vi "Teleop.vi"(10 "Match Info":T1={"Autonomous Elapsed Seconds"=0.0, "TeleOp Elapsed Seconds"=0.0, "Disabled Elapsed Seconds"=0.0, "Visited Autonomous"=FALSE, "Visited TeleOp"=FALSE, "Visited Disabled"=FALSE, "Autonomous Settings"={"Autonomous Style"=enum."Independent", "VI Refnum"=refnum}}, 11 "Call Context":T2) -> ()   [LabVIEW 2013]
doc: "This VI is called for each TeleOp packet received from the DS where the robot is not disabled. It is often used to read from the joysticks and update I/O or to update setpoints for timed control loops. It should complete and return within 20 milliseconds or it may miss DS packets."
uses:
  <vilib>/Rock Robotics/WPI/DriverStation/WPI_DriverStationDerivedRobotMode.ctl
  <vilib>/Rock Robotics/WPI/DriverStation/WPI_DriverStationMatch Info.ctl
  <vilib>/Rock Robotics/WPI/Relay/WPI_RelayValue.ctl
  <vilib>/Rock Robotics/WPI/Solenoid/WPI_SolenoidValue.ctl
  Robot Global Data.vi
  <vilib>/Rock Robotics/WPI/Solenoid/WPI_SolenoidSetEnum.vi
  <vilib>/Rock Robotics/WPI/Joystick/WPI_JoystickGetSetRefNum.vi
  <vilib>/Rock Robotics/WPI/RobotDrive/WPI_RobotDriveGetSetRefNum.vi
panel:
  out "Numeric 1":dbl(slide) scale=0.0..100.0
  out "Boolean 2":bool
  out "Boolean 1":bool
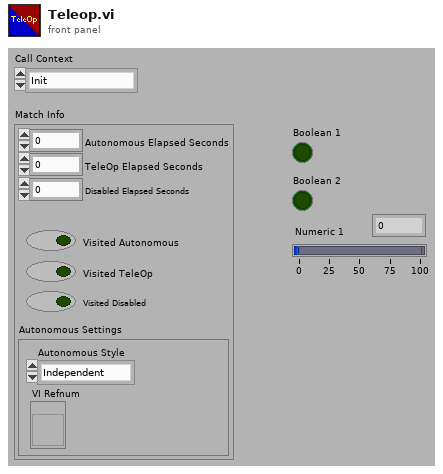
[diagram p1: front panel]
types:
  T1 = typedef "WPI_DriverStationMatch Info.ctl" = cluster{"Autonomous Elapsed Seconds":dbl, "TeleOp Elapsed Seconds":dbl, "Disabled Elapsed Seconds":dbl, "Visited Autonomous":bool, "Visited TeleOp":bool, "Visited Disabled":bool, "Autonomous Settings":cluster{"Autonomous Style":enum16{"Iterative", "Independent"}, "VI Refnum":refnum<vi>}}
  T2 = typedef "WPI_DriverStationDerivedRobotMode.ctl" = enum16{"Init", "Execute", "Stop"}
  T3 = typedef "WPI_SolenoidValue.ctl" = enum16{"Off", "On", "Forward", "Reverse"}
  T4 = typedef "WPI_RelayValue.ctl" = enum16{"Off", "On", "Forward", "Reverse"}
  T5 = typedef "WPI_JoystickDevRef.ctl" = cluster{"Device":T6}
  T6 = typedef "WPI_JoystickDeviceEnum.ctl" = enum16{"USB 1", "USB 2", "USB 3", "USB 4", "Kinect 1", "Kinect 2"}
  T7 = typedef "WPI_SolenoidDevRef.ctl" = cluster{"DevStatus":errorcluster, "Solenoid Module":T8, "Forward Solenoid Channel":T9, "Reverse Solenoid Channel":T9}
  T8 = typedef "FPGA_TypedefSolenoidModule.ctl" = enum16{"Solenoid Module 1", "Solenoid Module 2"}
  T9 = typedef "WPI_SolenoidChannel.ctl" = enum8{"Solenoid 1", "Solenoid 2", "Solenoid 3", "Solenoid 4", "Solenoid 5", "Solenoid 6", "Solenoid 7", "Solenoid 8", "Invalid"}
  T10 = typedef "WPI_JoystickButtonState.ctl" = cluster{"Button 1":bool, "Button 2":bool, "Button 3":bool, "Button 4":bool, "Button 5":bool, "Button 6":bool, "Button 7":bool, "Button 8":bool, "Button 9":bool, "Button 10":bool, "Button 11":bool, "Button 12":bool}
  T11 = cluster{"axis 1 (x)":dbl, "axis 2 (y)":dbl, "axis 3 (throttle)":dbl, "axis 4":dbl, "axis 5":dbl, "axis 6":dbl}
  T12 = typedef "WPI_RobotDriveDevRef.ctl" = cluster{"DevStatus":errorcluster, "Motors[]":T13[], "Square Inputs":bool, "Max Output":dbl, "Isochronous":bool}
  T13 = typedef "WPI_MotorControlDeviceRef.ctl" = cluster{"DeviceStatus":errorcluster, "Type":enum16{"PWM", "CAN"}, "PWM":cluster{"Digital Module":T14, "PWM Channel":T15, "DeadBand":T16}, "CAN":cluster{"Device Number":u8, "Control Mode":T17, "Semaphore":T18, "Max Vout":dbl}, "Invert":bool, "TransformRef":T19, "InvTransformRef":T19}
  T14 = typedef "FPGA_TypedefDigitalModule.ctl" = enum16{"Digital Module 1", "Digital Module 2"}
  T15 = typedef "FPGA_DIOPWMChannel.ctl" = enum8{"PWM 1", "PWM 2", "PWM 3", "PWM 4", "PWM 5", "PWM 6", "PWM 7", "PWM 8", "PWM 9", "PWM 10", "Invalid"}
  T16 = typedef "WPI_PWMDeadband.ctl" = cluster{"Name":string, "maxPositivePwm":i32, "minPositivePwm":i32, "centerPwm":i32, "maxNegativePwm":i32, "minNegativePwm":i32, "angularRange":u16}
  T17 = typedef "WPI_CANJaguar_ControlMode.ctl" = enum8{"Percent VBus", "Current", "Speed", "Position", "Voltage"}
  T18 = typedef "Semaphore RefNum" = refnum<k1>
  T19 = typedef "WPI_PWMTransform_ConPane.ctl" = refnum<vi>
  T20 = typedef "WPI_RelayDevRef.ctl" = cluster{"DevStatus":errorcluster, "Relay Channel":T21, "Digital Module":T14, "Relay Direction":T22}
  T21 = typedef "FPGA_DIORelayChannel.ctl" = enum8{"Relay 1", "Relay 2", "Relay 3", "Relay 4", "Relay 5", "Relay 6", "Relay 7", "Relay 8", "Invalid"}
  T22 = typedef "WPI_RelayDirection.ctl" = enum16{"Both directions", "Forward only", "Reverse only"}
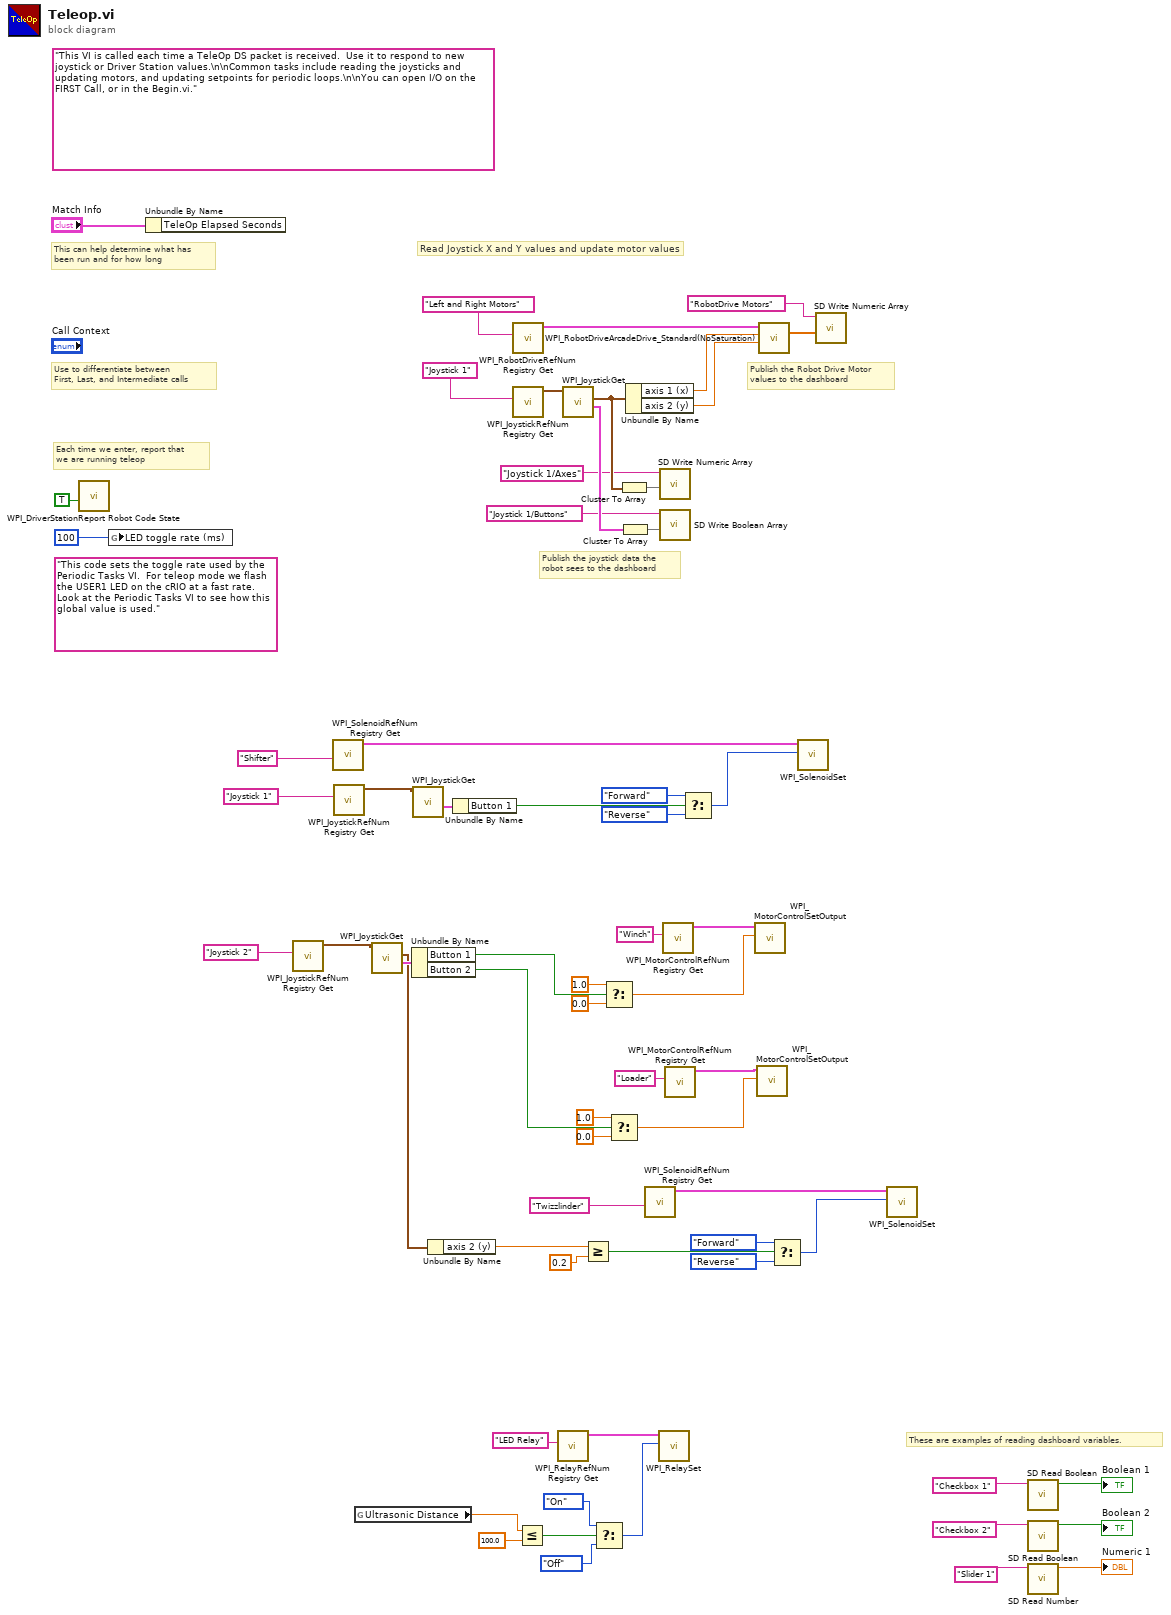
[diagram p0: block diagram]
diagram:
  (unwired) "This code sets the toggle rate used by the Periodic Tasks VI.  For teleop mode we flash the USER1 LED on the cRIO at a fast rate.  Look at the Periodic Tasks VI to see how this global value is used."
  (unwired) "This VI is called each time a TeleOp DS packet is received.  Use it to respond to new joystick or Driver Station values.\n\nCommon tasks include reading the joysticks and updating motors, and updating setpoints for periodic loops.\n\nYou can open I/O on the FIRST Call, or in the Begin.vi."
  # "These are examples of reading dashboard variables."
  # "Publish the Robot Drive Motor\nvalues to the dashboard"
  # "Publish the joystick data the\nrobot sees to the dashboard"
  # "Each time we enter, report that\nwe are running teleop"
  # "Use to differentiate between\nFirst, Last, and Intermediate calls"
  # "This can help determine what has\nbeen run and for how long"
  # "Read Joystick X and Y values and update motor values"
  n1 = call <vilib>:"WPI_DriverStationReport Robot Code State.vi"("TeleOp"=TRUE ("Autonomous")) -> ()  [unwired: 10 in, 1 out]
  n2 = global write "Robot Global Data.vi" "LED toggle rate (ms)"(u32 100 ("LED ms toggle rate")) -> ()
  n3 = Unbundle By Name("Match Info") -> ()  [unwired: 1 out]
  n4 = call <vilib>:"WPI_JoystickRefNum Registry Get.vi"("refnum name"="Joystick 2") -> ("JoystickDevRef"=w29:T5)  [unwired: 9 in, 1 out]
  n5 = call <vilib>:"WPI_SolenoidRefNum Registry Get.vi"("refnum name"="Shifter") -> ("SolenoidDevRef"=w35:T7)  [unwired: 9 in, 1 out]
  n6 = call <vilib>:"WPI_JoystickRefNum Registry Get.vi"("refnum name"="Joystick 1") -> ("JoystickDevRef"=w37:T5)  [unwired: 9 in, 1 out]
  n7 = global read "Robot Global Data.vi" "Ultrasonic Distance"() -> (w11:dbl)
  n8 = call <vilib>:"WPI_JoystickGet.vi"("JoystickDevRef"=w29) -> ("Buttons"=w28:T10, "Axes"=w9:T11)  [unwired: 4 in, 1 out]
  n9 = Unbundle By Name(w28) -> ("Button 1"=w23:bool, "Button 2"=w18:bool)
  n10 = call <vilib>:"WPI_JoystickGet.vi"("JoystickDevRef"=w37) -> ("Buttons"=w36:T10)  [unwired: 4 in, 2 out]
  n11 = Unbundle By Name(w9) -> ("axis 2 (y)"=w2:dbl)
  n12 = Unbundle By Name(w36) -> ("Button 1"=w31:bool)
  n13 = call <vilib>:"WPI_RobotDriveRefNum Registry Get.vi"("refnum name"="Left and Right Motors") -> ("RobotDriveDevRef"=w62:T12)  [unwired: 1 in, 9 out]
  n14 = call <vilib>:"WPI_JoystickRefNum Registry Get.vi"("refnum name"="Joystick 1") -> ("JoystickDevRef"=w58:T5)  [unwired: 1 in, 9 out]
  n15 = Less Or Equal?(x=w11, y=100.0) -> (x <= y?=w15:bool)
  n16 = call <vilib>:"WPI_RelayRefNum Registry Get.vi"("refnum name"="LED Relay") -> ("RelayDevRef"=w17:T20)  [unwired: 9 in, 1 out]
  n17 = call <vilib>:"WPI_JoystickGet.vi"("JoystickDevRef"=w58) -> ("Buttons"=w55:T10, "Axes"=w52:T11)  [unwired: 1 in, 4 out]
  n18 = Greater Or Equal?(x=w2, y=0.2) -> (x >= y?=w3:bool)
  n19 = Select(t=WPI_RelayValue."On" ("RelayValue"), s=w15, f=WPI_RelayValue."Off" ("RelayValue")) -> (s? t:f=w12:T4)
  n20 = Select(t=1.0, s=w23, f=0.0) -> (s? t:f=w19:dbl)
  n21 = Select(t=1.0, s=w18, f=0.0) -> (s? t:f=w20:dbl)
  n22 = Cluster To Array(cluster=w52) -> (array=w51:dbl[])
  n23 = Cluster To Array(cluster=w55) -> (array=w54:bool[])
  n24 = Unbundle By Name(w52) -> ("axis 1 (x)"=w61:dbl, "axis 2 (y)"=w60:dbl)
  n25 = call <vilib>:"WPI_SolenoidRefNum Registry Get.vi"("refnum name"="Twizzlinder") -> ("SolenoidDevRef"=w5:T7)  [unwired: 9 in, 1 out]
  n26 = call <vilib>:"WPI_RelaySet.vi"("RelayValue"=w12, "RelayDevRef"=w17) -> ()  [unwired: 8 in, 2 out]
  n27 = call <vilib>:"SD Write Numeric Array.vi"("Numeric Array"=w51, "Name"="Joystick 1/Axes") -> ()  [unwired: 8 in, 2 out]
  n28 = call <vilib>:"SD Write Boolean Array.vi"("Boolean Array"=w54, "Name"="Joystick 1/Buttons") -> ()  [unwired: 8 in, 2 out]
  n29 = call <vilib>:"WPI_MotorControlRefNum Registry Get.vi"("refnum name"="Winch") -> ("MotorControlDevRef"=w26:T13)  [unwired: 9 in, 1 out]
  n30 = call <vilib>:"WPI_MotorControlRefNum Registry Get.vi"("refnum name"="Loader") -> ("MotorControlDevRef"=w32:T13)  [unwired: 9 in, 1 out]
  n31 = Select(t=WPI_SolenoidValue."Forward", s=w31, f=WPI_SolenoidValue."Reverse" ("Value")) -> (s? t:f=w39:T3)
  n32 = call <vilib>:"WPI_MotorControlSetOutput.vi"("Output"=w19, "MotorControlDevRef"=w26) -> ()  [unwired: 7 in, 3 out]
  n33 = call <vilib>:"WPI_MotorControlSetOutput.vi"("Output"=w20, "MotorControlDevRef"=w32) -> ()  [unwired: 7 in, 3 out]
  n34 = call <vilib>:"WPI_RobotDriveArcadeDrive_Standard(NoSaturation).vi"("Y axis value"=w60, "X axis value"=w61, "RobotDriveDevRef"=w62) -> ("Motor Values"=w48:dbl[])  [unwired: 1 in, 7 out]
  n35 = Select(t=WPI_SolenoidValue."Forward", s=w3, f=WPI_SolenoidValue."Reverse" ("Value")) -> (s? t:f=w6:T3)
  n36 = call-poly <vilib>:"WPI_SolenoidSet.vi"("Value"=w39, "SolenoidDevRef"=w35) -> ()  [unwired: 1 in, 9 out]
  n37 = call <vilib>:"SD Write Numeric Array.vi"("Numeric Array"=w48, "Name"="RobotDrive Motors") -> ()  [unwired: 8 in, 2 out]
  n38 = call-poly <vilib>:"WPI_SolenoidSet.vi"("Value"=w6, "SolenoidDevRef"=w5) -> ()  [unwired: 1 in, 9 out]
  n39 = call <vilib>:"SD Read Boolean.vi"("Name"="Checkbox 1" ("refnum name")) -> ("Boolean"=→"Boolean 1":bool)  [unwired: 8 in, 2 out]
  n40 = call <vilib>:"SD Read Boolean.vi"("Name"="Checkbox 2" ("refnum name")) -> ("Boolean"=→"Boolean 2":bool)  [unwired: 8 in, 2 out]
  n41 = call <vilib>:"SD Read Number.vi"("Name"="Slider 1" ("refnum name")) -> ("Numeric"=→"Numeric 1":dbl)  [unwired: 8 in, 2 out]
